vi "SimpleGyro.vi"   [LabVIEW 2016, in "Moving Motor.lvrbt"]
uses:
  Moving Motor.lvrbt
  <vilib>/NXT/HiTechnic/HiTechnic Controls/HiTechnic Port.ctl
  <vilib>/NXT/Block Support/NXT_InputPort.ctl
types:
  T1 = typedef "HiTechnic Port.ctl" = cluster{"Port":T2, "MUX Port":u8}
  T2 = typedef "NXT_InputPort.ctl" = u32
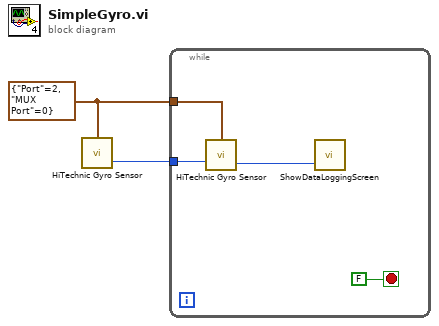
[diagram p0: block diagram]
diagram:
  w2 = T1 {"Port"=2, "MUX Port"=0} ("Port/MUX")
  n1 = call <vilib>:"HiTechnic Gyro Sensor.vi"("Port/MUX"=w2) -> ("Gyro Value"=w1:i16)  [unwired: 2 in, 1 out]
  n2 = while {
    tunnel: w2 -> [w6]
    tunnel: w1 -> [w5]
    stop <- FALSE stop-if-true
    n3 = call <vilib>:"HiTechnic Gyro Sensor.vi"("Offset"=w5, "Port/MUX"=w6) -> ("Gyro Value"=w4:i16)  [unwired: 1 in, 1 out]
    n4 = call <vilib>:"ShowDataLoggingScreen.vi"("Measured Value"=w4) -> ()  [unwired: 3 in, 1 out]
  }
